vi "oax_gsOrder Power Spectrum.vi"() -> ()   [LabVIEW 2017]
doc: "This is Order Analysis Toolkit demo VI."
uses:
  <vilib>/Waveform/WDTOps.llb/WDT Waveform Duration DBL.vi
  <vilib>/addons/Sound and Vibration/Order Analysis/Tach Process/SoundVib_TachProcess.lvlib
  <vilib>/addons/Sound and Vibration/Order Analysis/Resample Order Tracking/SoundVib_OrderTracking.lvlib
panel:
  out "averages completed":dbl
  out "averaging done?":bool
  in  "restart averaging (F)":bool
  in  "averaging parameters":T1={"averaging mode"=enum."No averaging", "weighting mode"=enum."Exponential", "number of averages"=10, "linear mode"=enum."One shot"} {"number of averages" min=1 step=1}
  in  "block size":i32=1024 min=2
  in  "window type":u32(ring)=1 items=["None"=0, "Hanning"=1, "Hamming"=2, "Blackman-Harris"=3, "Exact Blackman"=4, "Blackman"=5, "Flat Top"=6, "4 Term B-Harris"=7, "7 Term B-Harris"=8, "Low Sidelobe"=9, "Gaussian"=62]
  in  "dB on (T)":bool=TRUE
  out "Power spectrum":T2(graph)
  in  "Select Data":i32(listbox)
  in  "STOP":bool
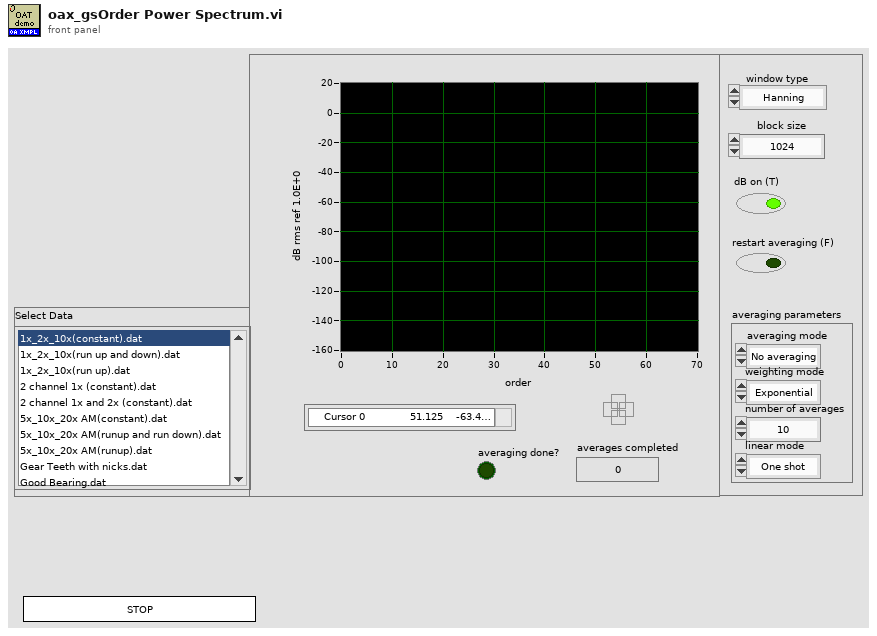
[diagram p1: front panel]
types:
  T1 = cluster{"averaging mode":enum16{"No averaging", "Vector averaging", "RMS averaging", "Peak hold"}, "weighting mode":enum16{"Linear", "Exponential"}, "number of averages":u32, "linear mode":enum16{"One shot", "Auto restart"}}
  T2 = cluster{"order 0":dbl, "delta order":dbl, "magnitude":dbl[]}
  T3 = typedef "SoundVib_TachProcess.lvlib/speed profile.ctl" = cluster{"time [s]":dbl[], "speed [RPM]":dbl[]}
  T4 = typedef "svc_Resampled Channel Info.ctl" = cluster{"channel name":string, "description":string, " channel info":T5}
  T5 = typedef "svc_Channel Info.ctl" = cluster{"sensor sensitivity":dbl, "engineering units":T6, "dB reference":dbl, "custom label":string, "weighting filter":T7, "pregain":dbl}
  T6 = typedef "svc_Engineering Units Text Ring.ctl" = u16
  T7 = typedef "svc_Weighting Filter Text Ring.ctl" = u16
  T8 = cluster{"pulse / rev":i32, "threshold (auto)":dbl, "slope (Rising)":u16}
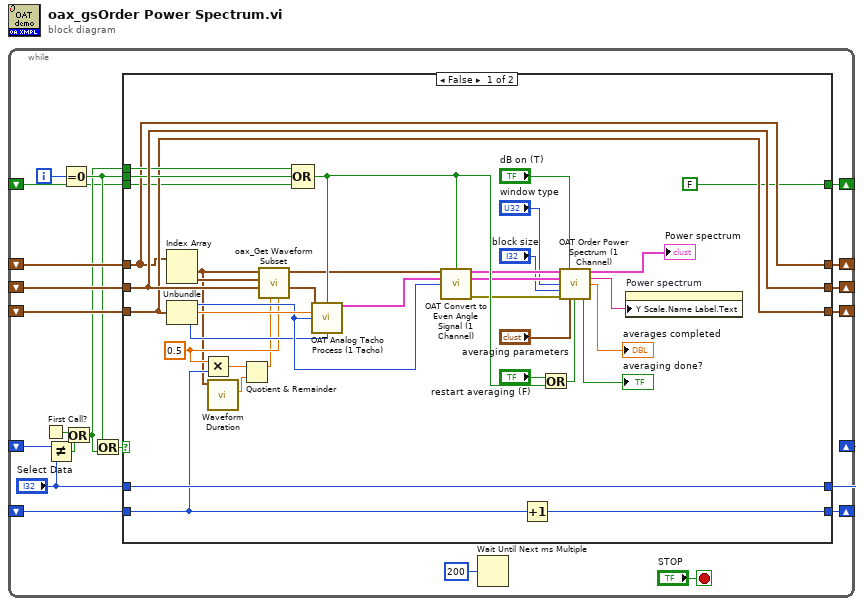
[diagram p0: block diagram]
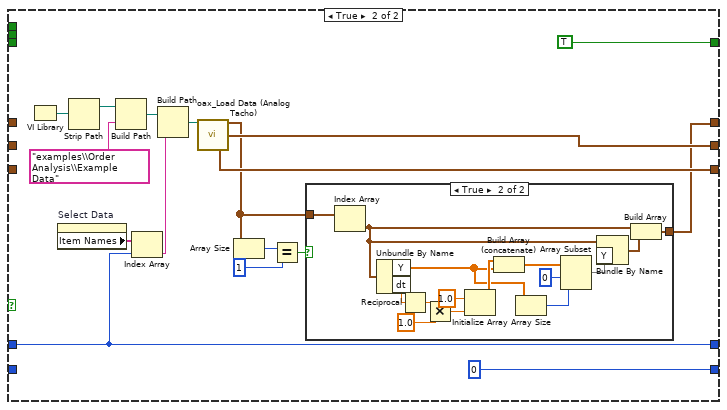
[diagram p2: hidden frame]
diagram:
  n1 = while {
    shift-right: [w17] -> _
    shift-left: _ -> [w18]
    shift-right: [w15] -> _
    shift-left: _ -> [w21]
    shift-right: [w14] -> _
    shift-left: _ -> [w19]
    shift-right: [w13] -> _
    shift-left: _ -> [w12]
    shift-right: [w3] -> _
    shift-left: _ -> [w4]
    shift-right: [w2] -> _
    shift-left: _ -> [w1]
    i -> [w11]
    stop <- "STOP" stop-if-true
    n2 = First Call?() -> (First Call?: T/F=w7:bool)
    n3 = Not Equal?(x=w18, y="Select Data") -> (x != y?=w6:bool)
    n4 = Equal To 0?(x=w11) -> (x = 0?=w10:bool)
    n5 = Or(x=w7, y=w6) -> (x .or. y?=w5:bool)
    n6 = Or(x=w10, y=w5) -> (x .or. y?=w9:bool)
    n7 = case shown="False" w9 {
      tunnel: w21 -> [w37 _]
      tunnel: w19 -> [w55 _]
      tunnel: [w56 w73] -> w17
      tunnel: "Select Data" -> [w56 w73]
      tunnel: [w37 w58] -> w15
      tunnel: [w55 w71] -> w14
      tunnel: [w48 w70] -> w13
      tunnel: w12 -> [w48 _]
      tunnel: w5 -> [w53 _]
      tunnel: w10 -> [w52 _]
      tunnel: w4 -> [w42 _]
      tunnel: [w44 0] -> w3
      tunnel: [FALSE TRUE] -> w2
      tunnel: w1 -> [w36 _]
      frame False {
        w43 = 0.5 ("y")
        n8 = Index Array(array=w37) -> (element #1=w41:waveform(dbl), element #2=w49:waveform(dbl))  [unwired: 2 in]
        n9 = Unbundle(w48) -> ("pulse / rev"=w46:i32, "threshold (auto)"=w47:dbl, "slope (Rising)"=w45:u16)
        n10 = Multiply(x=w43, y=w42) -> (x*y=w39:dbl)
        n11 = call-poly <vilib>:"Waveform Duration.vi"("waveform in"=w41) -> ("duration"=w40:dbl)  [unwired: 8 in, 2 out]
        n12 = Quotient & Remainder(x=w39, y=w40) -> (x-y*floor(x/y)=w38:dbl)  [unwired: 1 out]
        n13 = call <vilib>:"oax_Get Waveform Subset.vi"("duration"=w43, "start index"=w38, "Tach Signal"=w55, "Vibration Signal Y"=w49, "Vibration Signal X"=w41) -> ("Tach Signal out"=w54:waveform(dbl), "Vibration Signal X out"=w50:waveform(dbl))  [unwired: 3 in, 2 out]
        n14 = Compound Arithmetic op=OR(w53, w52, w36) -> (w51:bool)
        n15 = call <vilib>:"OAT Analog Tacho Process (1 Tacho).vi"("analog tacho signal"=w54, "reset? (F)"=w51, "threshold (auto)"=w47, "pulse/revolution (1)"=w46, "slope (Rising)"=w45) -> ("speed profile"=w57:T3)  [unwired: 6 in, 4 out]
        n16 = call <vilib>:"OAT Convert to Even Angle Signal (1 Channel).vi"("scaled signal [EU]"=w50, "reset? (F)"=w51, "speed profile"=w57, "pulse/revolution (1)"=w46) -> ("even-angle signal"=w33:cluster{"r0":dbl, "dr":dbl, "Y":dbl[]}, "even-angle channel info"=w32:T4, "error out"=w34:errorcluster)  [unwired: 7 in, 2 out]
        n17 = Increment(x=w42) -> (x+1=w44:i32)
        n18 = Or(x="restart averaging (F)", y=w51) -> (x .or. y?=w25:bool)
        n19 = call <vilib>:"OAT Order Power Spectrum (1 Channel).vi"("even-angle signal"=w33, "dB on? (T)"="dB on (T)", "even-angle channel info"=w32, "window"="window type", "block size"="block size", "error in (no error)"=w34, "averaging parameters"="averaging parameters", "restart averaging? (F)"=w25) -> ("order power spectrum"=→"Power spectrum":T2, "unit label"=w24:string, "averages completed"=→"averages completed":dbl, "averaging done?"=→"averaging done?":bool)  [unwired: 1 in, 3 out]
        n20 = property on="Power spectrum" class="WFGraph (strict)"("Y Scale.Name Label.Text"=w24) -> ()  [unwired: 2 in, 2 out]
      }
      frame True {
        n21 = VI Library() -> (path=w66:path)
        n22 = property on="Select Data" class="LstBox (strict)"() -> ("Item Names"=w74:string[])  [unwired: 2 in, 2 out]
        n23 = Strip Path(path=w66) -> (stripped path=w65:path)  [unwired: 1 out]
        n24 = Build Path(base path=w65, name or relative path="examples\\Order Analysis\\Example Data") -> (appended path=w69:path)
        n25 = Index Array(array=w74, index=w73) -> (element=w68:string)
        n26 = Build Path(base path=w69, name or relative path=w68) -> (appended path=w67:path)
        n27 = call <vilib>:"oax_Load Data (Analog Tacho).vi"("Data Path In"=w67) -> ("vibration data"=w59:waveform(dbl)[], "analog tacho signal"=w71:waveform(dbl), "tacho info"=w70:T8)  [unwired: 8 in, 4 out]
        n28 = Array Size(array=w59) -> (size(s)=w62:i32)
        n29 = Equal?(x=w62, y=1) -> (x = y?=w60:bool)
        n30 = case shown="True" w60 {
          tunnel: w59 -> [w75 w90]
          tunnel: [w75 w89] -> w58
          frame False {
          }
          frame True {
            n31 = Index Array(array=w90) -> (element=w88:waveform(dbl))  [unwired: 1 in]
            n32 = Unbundle By Name(w88) -> ("Y"=w77:dbl[], "dt"=w86:dbl)
            n33 = Reciprocal(x=w86) -> (1/x=w85:dbl)
            n34 = Multiply(x=w85, y=1.0) -> (x*y=w83:dbl)
            n35 = Initialize Array(1.0 ("element"), w83) -> (w79:dbl[])
            n36 = Build Array (concatenate)(w79, w77) -> (w81:dbl[])
            n37 = Array Size(array=w77) -> (size(s)=w78:i32)
            n38 = Array Subset(array=w81, index=0, length=w78) -> (w76:dbl[])
            n39 = Bundle By Name(cluster=w88, "Y"=w76) -> (w87:waveform(dbl))
            n40 = Build Array(w88, w87) -> (w89:waveform(dbl)[])
          }
        }
      }
    }
    n41 = Wait Until Next ms Multiple(millisecond multiple=u32 200) -> ()  [unwired: 1 out]
  }
